vi "UE9 Stream Simple Example.vi"() -> ()   [LabVIEW 2021]
panel:
  out "UD Backlog [%]":dbl format="%.2f"
  out "Actual Scan Rate (Hz)":dbl=1000.0 format="%.3f"
  out "# Scans Read":i32
  out "# of iterations":i32
  out "Data":dbl[][](array[numeric]) format="%.3f"
  in  "Scan Rate (Hz)":dbl=1000.0 format="%.3f"
  in  "stop":bool
  out "Error Message":string
  # "This example streams from AIN0-AIN3,\nusing the first found USB UE9."
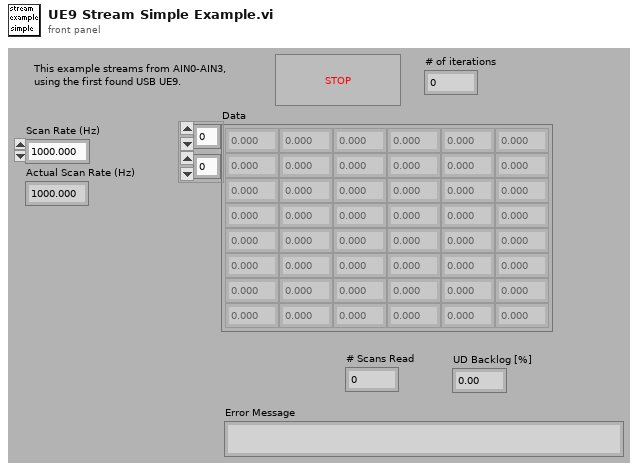
[diagram p1: front panel]
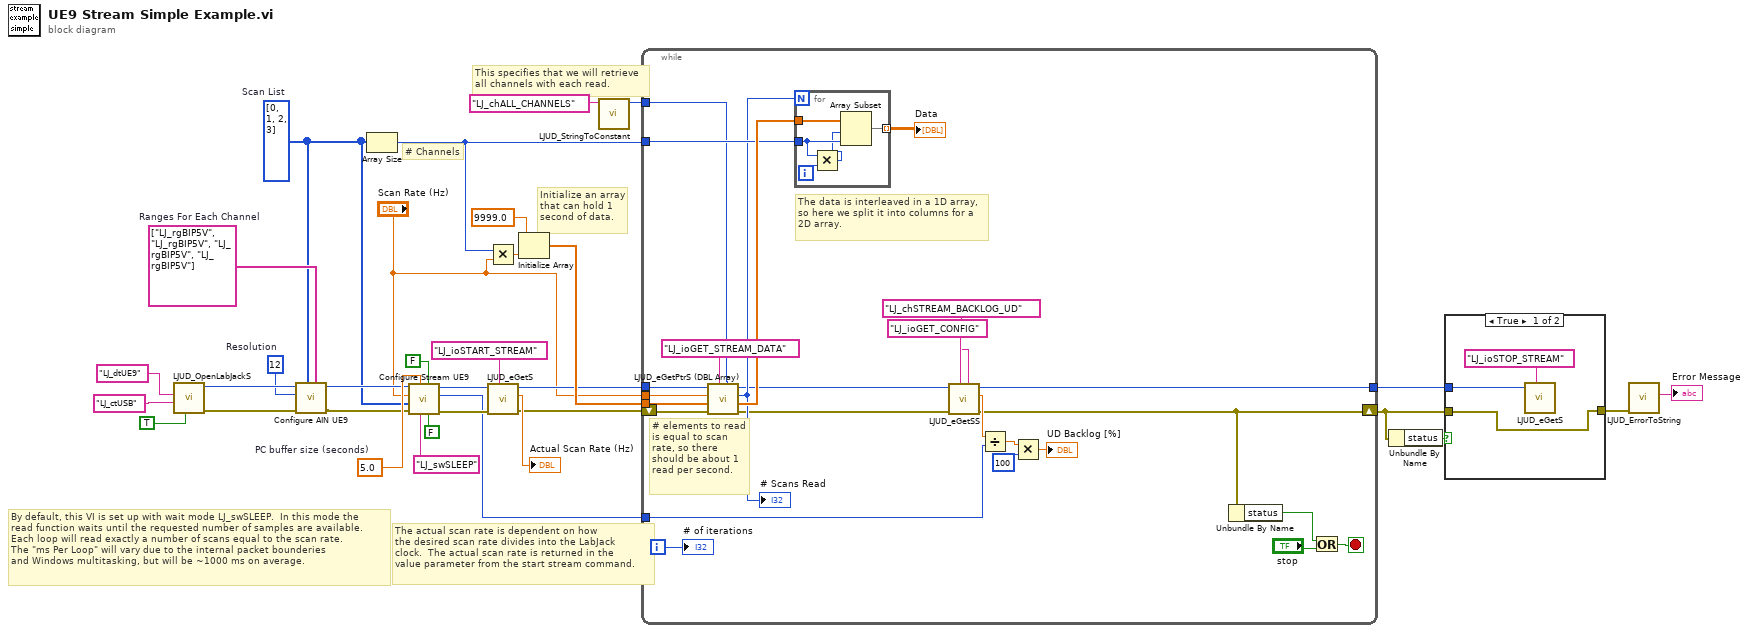
[diagram p0: block diagram]
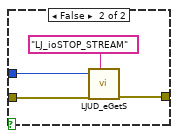
[diagram p2: hidden frame]
diagram:
  w7 = 12  # Resolution
  w8 = i32[] [0, 1, 2, 3]  # Scan List
  w9 = string[] ["LJ_rgBIP5V", "LJ_rgBIP5V", "LJ_rgBIP5V", "LJ_rgBIP5V"]  # Ranges For Each Channel
  w22 = 5.0  # PC buffer size (seconds)
  # "Initialize an array\nthat can hold 1\nsecond of data."
  # "# Channels"
  # "This specifies that we will retrieve\nall channels with each read."
  # "The actual scan rate is dependent on how\nthe desired scan rate divides into the LabJack\nclock.  The actual scan rate is returned in the\nvalue parameter from the start stream command."
  # "By default, this VI is set up with wait mode LJ_swSLEEP.  In this mode the\nread function waits until the requested number of samples are available.\nEach loop will read exactly a number of scans equal to the scan rate.\nThe \"ms Per Loop\" will vary due to the internal packet bounderies\nand Windows multitasking, but will be ~1000 ms on average."
  n1 = call "LJUD_OpenLabJackS.vi"("FirstFound"=TRUE, "ConnectionType"="LJ_ctUSB", "DeviceType"="LJ_dtUE9") -> ("error out"=w16:errorcluster, "Handle"=w15:i32)  [unwired: 6 in, 1 out]
  n2 = call "Configure AIN UE9.vi"("Ranges"=w9, "Channels"=w8, "error in"=w16, "Resolution"=w7, "Handle In"=w15) -> ("error out"=w18:errorcluster, "Handle Out"=w17:i32)  [unwired: 5 in]
  n3 = Array Size(array=w8) -> (size(s)=w27:i32)
  n4 = call "Configure Stream UE9.vi"("External Scan Trigger"=FALSE, "Scan Clock Output"=FALSE, "Wait Mode"="LJ_swSLEEP" ("Wait Mode (2)"), "PC buffer size (seconds)"=w22, "error in"=w18, "Scan List"=w8, "Scan Rate (Hz)"="Scan Rate (Hz)", "Handle In"=w17) -> ("error out"=w31:errorcluster, "PC buffer size (samples)"=w1:i32, "Handle Out"=w32:i32)  [unwired: 1 in]
  n5 = Multiply(x=w27, y="Scan Rate (Hz)") -> (x*y=w30:dbl)
  n6 = call "LJUD_eGetS.vi"("IOType"="LJ_ioSTART_STREAM", "error in"=w31, "Handle In"=w32) -> ("error out"=w2:errorcluster, "Value Read"=→"Actual Scan Rate (Hz)":dbl, "Handle Out"=w14:i32)  [unwired: 6 in]
  n7 = Initialize Array(9999.0, w30) -> (w28:dbl[])
  n8 = call "LJUD_StringToConstant.vi"("String"="LJ_chALL_CHANNELS") -> ("Constant Number"=w10:i32)  [unwired: 9 in, 1 out]
  n9 = while {
    tunnel: w1 -> [w34]
    shift-left: w2 -> [w45]
    shift-right: [w36] -> w3
    tunnel: w10 -> [w48]
    tunnel: [w35] -> w25
    tunnel: w27 -> [w51]
    tunnel: w28 -> [w54]
    tunnel: "Scan Rate (Hz)" -> [w52]
    tunnel: w14 -> [w56]
    i -> [w50]
    stop <- w47 stop-if-true
    # "The data is interleaved in a 1D array,\nso here we split it into columns for a\n2D array."
    # "# elements to read\nis equal to scan\nrate, so there\nshould be about 1\nread per second."
    n10 = call "LJUD_eGetPtrS (DBL Array).vi"("Channel"=w48, "IOType"="LJ_ioGET_STREAM_DATA", "error in"=w45, "DBL Array Write"=w54, "Value"=w52, "Handle In"=w56) -> ("error out"=w37:errorcluster, "DBL Array Read"=w53:dbl[], "Value"=w46:i32, "Handle Out"=w38:i32)  [unwired: 2 in]
    "# Scans Read" <- w46
    n11 = for {
      N: w46 -> [_]
      tunnel: w53 -> [w63]
      tunnel: w51 -> [w62]
      tunnel: [w59] -> w49 mode=indexing
      i -> [w61]
      n12 = Multiply(x=w62, y=w61) -> (x*y=w60:i32)
      n13 = Array Subset(array=w63, index=w60, length=w62) -> (w59:dbl[])
    }
    "Data" <- w49
    n14 = call "LJUD_eGetSS.vi"("Channel"="LJ_chSTREAM_BACKLOG_UD", "IOType"="LJ_ioGET_CONFIG", "error in"=w37, "Handle In"=w38) -> ("error out"=w36:errorcluster, "Value Read"=w40:dbl, "Handle Out"=w35:i32)  [unwired: 5 in]
    n15 = Divide(x=w40, y=w34) -> (x/y=w41:dbl)
    n16 = Multiply(x=w41, y=100) -> (x*y=→"UD Backlog [%]":dbl)
    n17 = Unbundle By Name(w36) -> ("status"=w57:bool)
    n18 = Or(x=w57, y="stop") -> (x .or. y?=w47:bool)
    "# of iterations" <- w50
  }
  n19 = Unbundle By Name(w3) -> ("status"=w12:bool)
  n20 = case shown="True" w12 {
    tunnel: w25 -> [w65 w69]
    tunnel: [w64 w68] -> w24
    tunnel: w3 -> [w64 w67]
    frame True {
      n21 = call "LJUD_eGetS.vi"("IOType"="LJ_ioSTOP_STREAM", "Handle In"=w65) -> ()  [unwired: 7 in, 3 out]
    }
    frame False {
      n22 = call "LJUD_eGetS.vi"("IOType"="LJ_ioSTOP_STREAM", "error in"=w67, "Handle In"=w69) -> ("error out"=w68:errorcluster)  [unwired: 6 in, 2 out]
    }
  }
  n23 = call "LJUD_ErrorToString.vi"("error in"=w24) -> ("String"=→"Error Message":string)  [unwired: 10 in]
